vi "format set indent.vi"(8 "error in (no error)":errorcluster, 10 "level":u8, 11 "format":u32) -> (0 "error out":errorcluster)   [LabVIEW 2015, in "xlsxwriter.lvlib"]
doc: "void format_set_indent(lxw_format format, uint8_t level);"
uses:
  xlsxwriter.lvlib
  xlsxwriter.dll
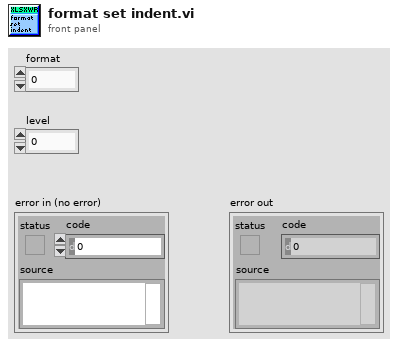
[diagram p1: front panel]
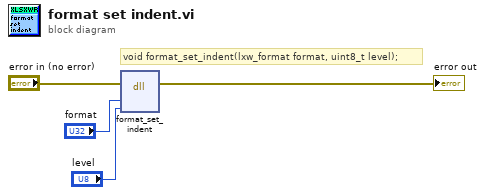
[diagram p0: block diagram]
diagram:
  # "void format_set_indent(lxw_format format, uint8_t level);"
  n1 = dll-call lib="C:/Users/WDAGUtilityAccount/Desktop/lv_vis_added_cell/xlsxwriter.*" fn="format_set_indent"(error in="error in (no error)", "format"="format", "level"="level") -> (error out=→"error out":errorcluster)  [unwired: 5 in, 1 out]
